vi "duty.vi"() -> ()   [LabVIEW 2017]
panel:
  out "Duty Cycle":dbl
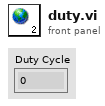
[diagram p1: front panel]
diagram:
